vi "Insert into Subpanel.vi"(8 "error in (no error)":errorcluster, 10 "SubPanel":refnum<vi>, 11 "Standard VI Type in":refnum<class "Standard VI Type.lvclass">) -> (0 "error out":errorcluster, 3 "Standard VI Type out":refnum<class "Standard VI Type.lvclass">)   [LabVIEW 2020, in "Peek Window.lvlib" / "Standard VI Type.lvclass"]
uses:
  Standard VI Type.lvclass
  Standard VI Type.lvclass/Standard VI Type.ctl
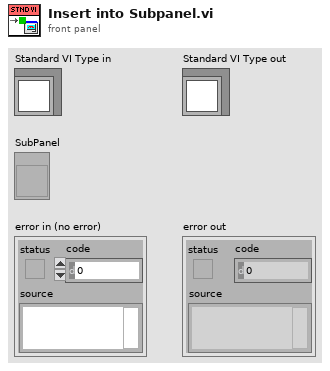
[diagram p1: front panel]
types:
  T1 = enum8{"Enabled", "Disabled", "Disabled and Grayed Out"}
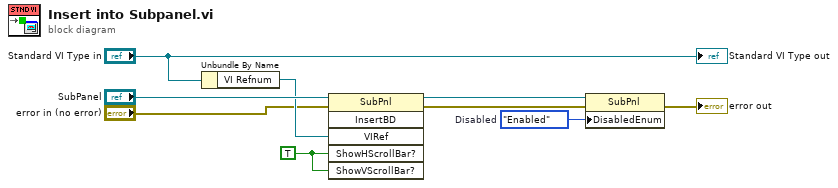
[diagram p0: block diagram]
diagram:
  w4 = T1."Enabled"  # Disabled
  w8 = TRUE ("ShowHScrollBar")
  n1 = Unbundle By Name("Standard VI Type in") -> ("VI Refnum"=w6:refnum<vi>)
  n2 = invoke on="Invoke Node" class="SubPnl" method="InsertBD"(reference="SubPanel", error in="error in (no error)", "VIRef"=w6, "ShowHScrollBar?"=w8, "ShowVScrollBar?"=w8) -> (reference out=w3:refnum<vi>, error out=w2:errorcluster)  [unwired: 1 in, 4 out]
  n3 = property class="SubPnl"(reference=w3, error in=w2, "DisabledEnum"=w4) -> (error out=→"error out":errorcluster)  [unwired: 1 out]
  "Standard VI Type out" <- "Standard VI Type in"
